vi "Dashboard Main.vi"() -> ()   [LabVIEW 2014]
uses:
  <vilib>/event_ctls.llb/eventvkey.ctl
  <vilib>/Rock Robotics/WPI/Dashboard/WPI_DashboardLogging Global.vi
  <vilib>/Rock Robotics/Network Tables/SD Read Number.vi
  <vilib>/Rock Robotics/Network Tables/SD Read Boolean.vi
  <vilib>/Rock Robotics/Network Tables/SD Write Number.vi
  <vilib>/Utility/config.llb/Write Key (String).vi
  <vilib>/Utility/config.llb/Write Key (I32).vi
  <vilib>/Utility/config.llb/NI_LVConfig.lvlib
panel:
  in  "TCP":refnum<k5>
  in  "Rec Mode":enum32{"Stop", "Record", "Playback"}(radio)
  in  "Vision":u16(ring) items=["Camera Off", "USB Camera SW", "USB Camera HW", "IP Camera"]
  out "Camera IP":string
  out "Image Message":string="Timeout in Camera Communications"
  in  "Dashboard Tab":T1(tab)
  out "Gauge":dbl(knob) scale=-0.8..0.8
  out "LatchContainerState":bool
  out "LatchLatchState":bool
  out "LatchLinkState":bool
  out "GateCylState":bool
  out "LiftCurrentHeight":dbl(slide) scale=0.0..1500.0
  out "LiftRequestedHeight":dbl(slide) scale=0.0..1500.0
  in  "ChassisSpeedDivider":dbl(slide) scale=1.25..2.0
  out "Accel":T2(graph)
  in  "Camera Settings":T3={"Frame Rate"=30, "Compression"=30, "Size"=1} {"Frame Rate" scale=1.0..30.0; "Size" items=["640x480", "320x240", "160x120"]}
  out "Mode":T4(ring)=enum."Auto Disabled"
  in  "DB Camera Config":bool
  out "fps":dbl format="%#.1g"
  out "Mbps":dbl format="%#.1g"
  out "Mbps 2":bool
  out "LiftData":T2(graph)
  in  "Test Slider":dbl(slide) scale=0.0..100.0 scale format="%#_3g"
  in  "On/Off":bool caption="Solenoid"
  in  "Test Name":u16(ring) items=["Select the test to run...", "Example Test", "-------------------------------", "List of tests is built in robot code.", "Replace with your own automated tests."]
  in  "Test Tree":string(tree)
  in  "Motor":cluster{"Value":dbl, "Enable":bool} {"Value" scale=-1.0..1.0 scale format="%#_3g"}
  out "Progress":T5 {"Test Progress" scale=0.0..100.0}
  in  "Rev/Fwd":cluster{"Forward":bool, "Reverse":bool}
  in  "Test Ring":u16(ring) items=["Monochrome", "Color"]
  in  "Listbox":i32(listbox)
  out "Tree":string(tree)
  out "Camera Image":T6(plugin-control)
  out "Boolean":bool
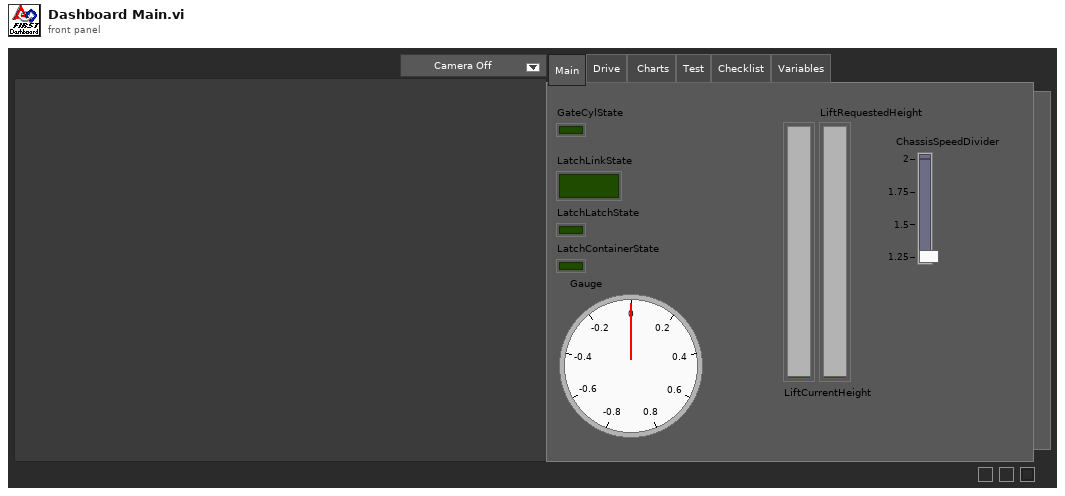
[diagram p1: front panel]
types:
  T1 = enum32{"Main", "Drive", " Charts", "Test", "Checklist", "Variables"}
  T2 = cluster{"Numeric":dbl, "Numeric":dbl, "Numeric":dbl}
  T3 = cluster{"Frame Rate":i32, "Compression":i32, "Size":u16}
  T4 = enum8{"Tele-Op Disabled", "Tele-Op Enabled", "Auto Disabled", "Auto Enabled", "Test Disabled", "Test Enabled", "Disconnected", "No Code", "E-Stop"}
  T5 = cluster{"Test Progress":u8, "Test Progress Text":string}
  T6 = typedef "IMAQ Image.ctl" = refnum<image>
  T7 = enum32{"Drive", "Basic", "Custom", "Test", "Checklist", "Variables"}
  T8 = typedef "Image Type" = u32
  T9 = cluster{"Camera Image":refnum<vi>, "Dashboard Tab":refnum<vi>, "Boolean":refnum<vi>, "Vision":refnum<vi>, "Rec Mode":refnum<vi>, "Test Slider":refnum<vi>, "On/Off ":refnum<vi>, "Test Ring":refnum<vi>, "Rev/Fwd":refnum<vi>, "Test Name":refnum<vi>, "Motor":refnum<vi>, "Progress":refnum<vi>, "CheckList":refnum<vi>, "Tree":refnum<vi>, "Test Tree":refnum<vi>}
  T10 = cluster{"Error Strings":string, "Disable Counts":cluster{u16, u16}, "Rail Faults":cluster{u16, u16, u16}, "Robot IP":string, "DB Mode":u8, "Event Info":cluster{"Name":string, "Type":u8, "Number":u16, "Replay":u8}, "Camera Addr":string}
  T11 = cluster{"Storage":cluster{"Disk Free":u64, "RAM Block":u32, "RAM free":u32}, "CPU Utilization":cluster{"CPU % ISR":sgl, "CPU % Time Crit":sgl, "CPU % Timed Str":sgl, "CPU % High":sgl, "CPU % Above":sgl, "CPU % Normal":sgl, "CPU % Low":sgl}, "CAN":cluster{"% Bus Utilization":sgl, "Bus Off Cnt":u32, "TX_FIFO Full Cnt":u32, "Receive Error Cnt":u8, "Transmit Error Cnt":u8}, "HID":cluster{"HID Outputs":u32, "Rumble Low":u16, "Rumble High":u16}[]}
  T12 = cluster{"Status bits":cluster{"Test Mode":bool, "Autonomous":bool, "Enabled":bool, "Code Start":bool, "Brownout":bool, "Reserved 2":bool, "Reserved 3":bool, "E-Stop":bool}, "Code Trace":cluster{"Disabled":bool, "TeleOp":bool, "Auto":bool, "Test":bool}, "Controller Type":enum16{"unknown", "cRIO", "roboRio"}, "Code?":enum16{"unknown", "noCode", "code"}, "Battery V":dbl}
  T13 = cluster{"Control Bits":cluster{"TestMode":bool, "Autonomous":bool, "Enabled":bool, "FMS Present":bool, bool, bool, bool, "E-Stop":bool}, "Team Station ":u8, "Countdown":sgl, "Joystick Values":cluster{"Axes":dbl[], "Buttons":bool[], "POVs":i16[]}[]}
  T14 = typedef "NI_LVConfig.lvlib/Config Data RefNum.ctl" = refnum<k1>
  T15 = cluster{"Operation":enum16{"Update", "Clear"}, "Color Box":u32}[]
  T16 = typedef "eventvkey.ctl" = enum16{"ASCII", "Enter", "Return", "Shift", "Ctrl", "Alt", "Cmd", "Opt", "Caps", "NumLock", "Clear", "Break", "Up", "Down", "Left", "Right", "Insert", "Delete", "Home", "End", "PageUp", "PageDown", "Escape", "Help", "Pause", "ScrollLock", "F1", "F2", "F3", "F4", "F5", "F6", "F7", "F8", "F9", "F10", "F11", "F12", "F13", "F14", "F15", "F16", "F17", "F18", "F19", "F20", "F21", "F22", "F23", "F24", "Play", "VolumeUp", "VolumeDown", "Mute", "Two Byte Char"}
  T17 = cluster{"Image Size":bool, "Image Type":bool, "Pixel Value":bool, "ROI Information":bool, "Zoom Factor":bool}
  T18 = enum8{"Enabled", "Disabled", "Disabled and Grayed Out"}
  T19 = cluster{"Operation":enum16{"Update", "Clear"}, "Color Box":u32}
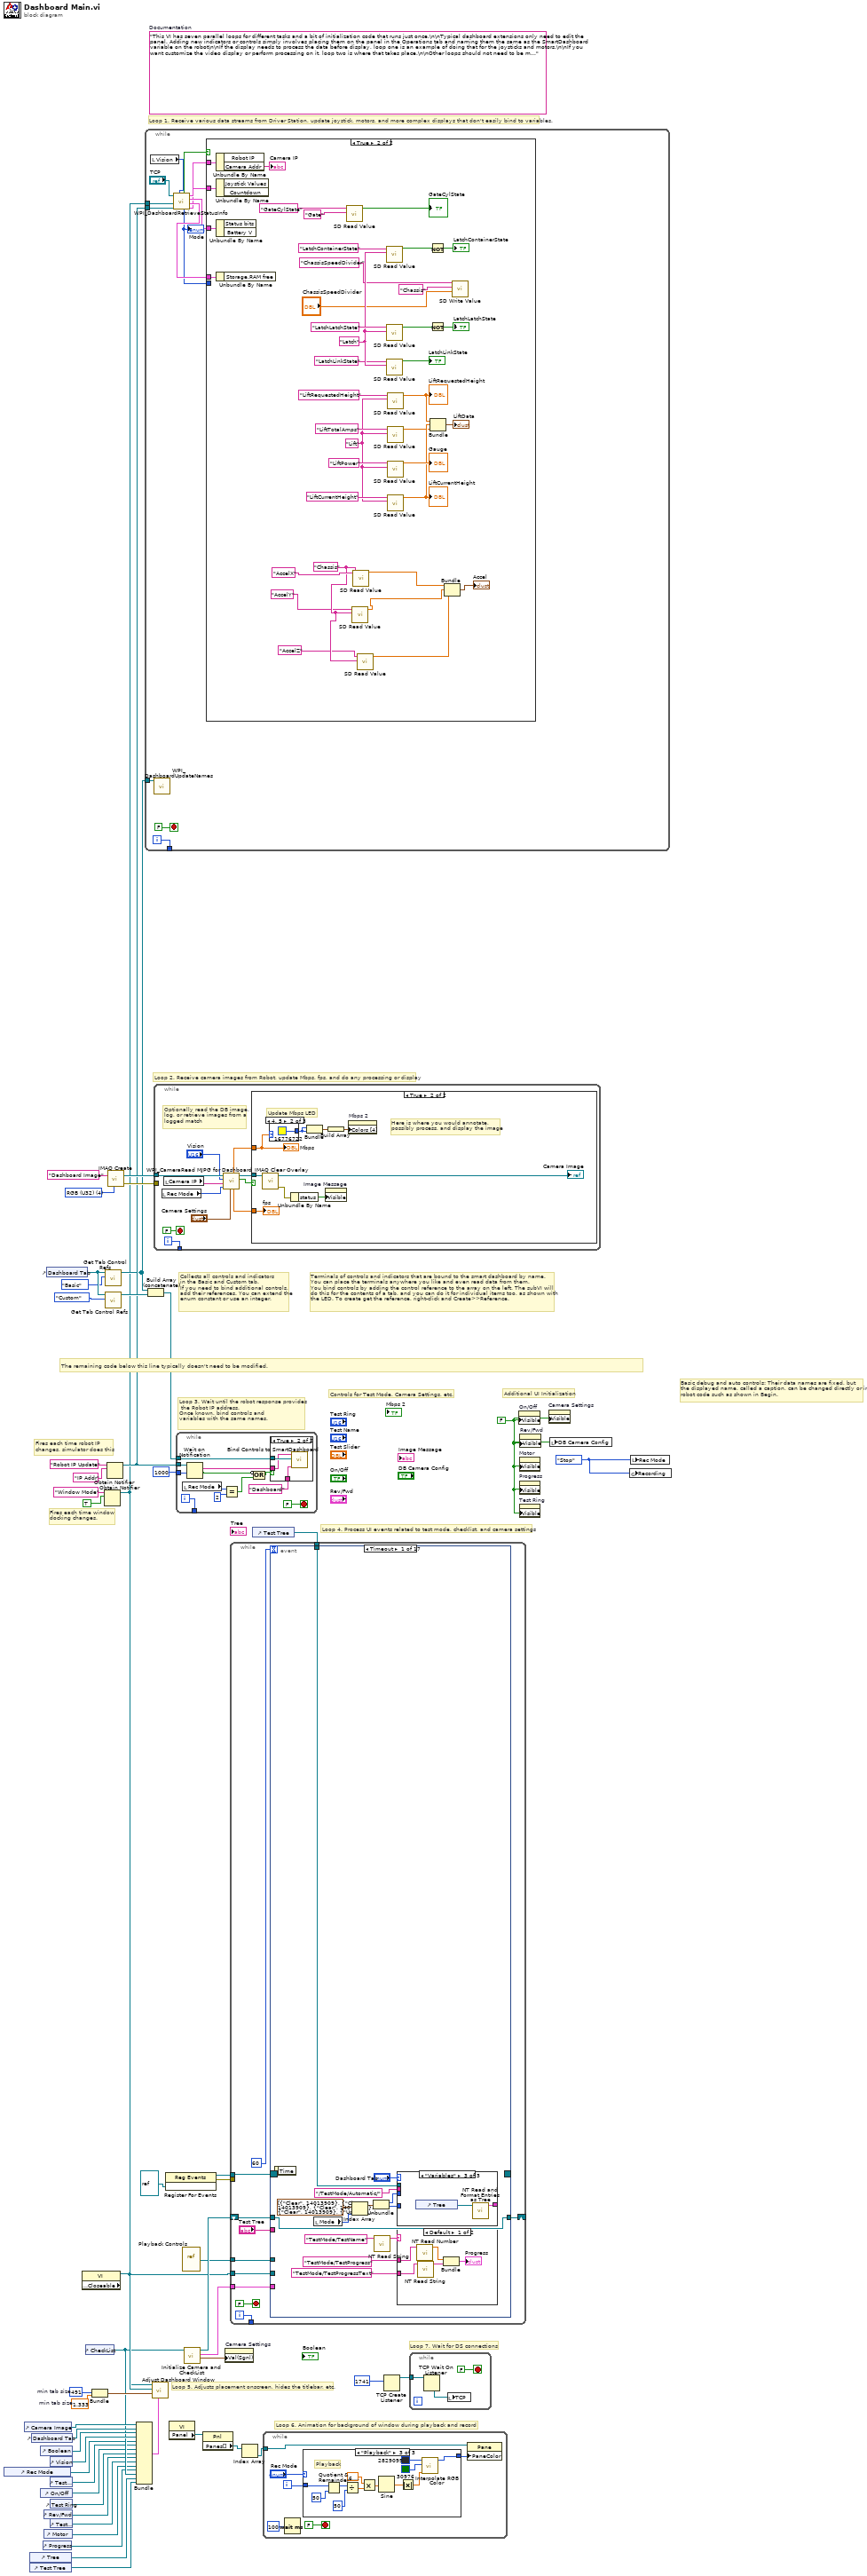
[diagram p0: block diagram]
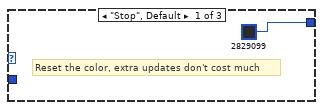
[diagram p3: hidden frame]
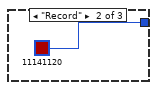
[diagram p4: hidden frame]
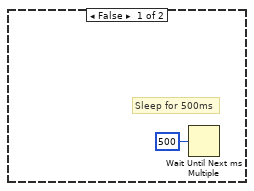
[diagram p6: hidden frame]
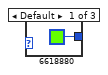
[diagram p7: hidden frame]
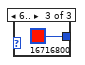
[diagram p8: hidden frame]
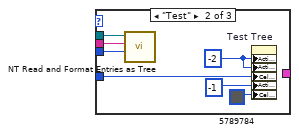
[diagram p10: hidden frame]
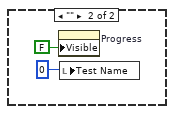
[diagram p11: hidden frame]
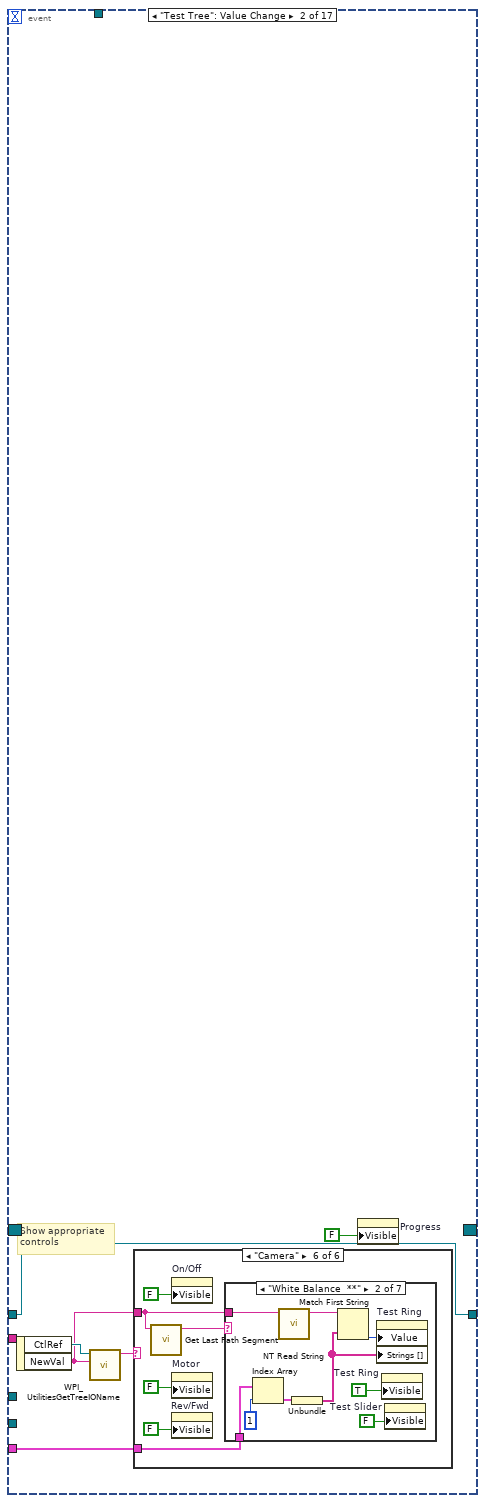
[diagram p12: hidden frame]
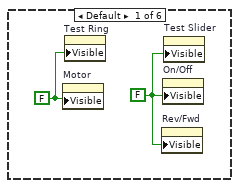
[diagram p13: hidden frame]
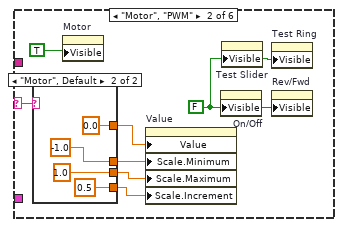
[diagram p14: hidden frame]
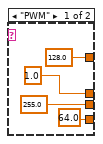
[diagram p15: hidden frame]
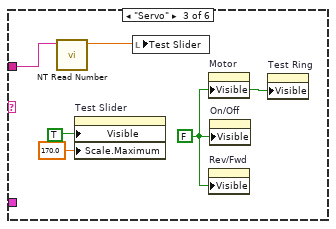
[diagram p16: hidden frame]
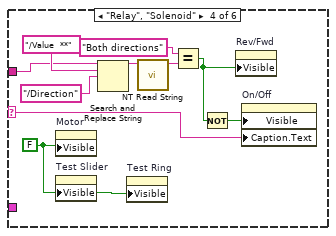
[diagram p17: hidden frame]
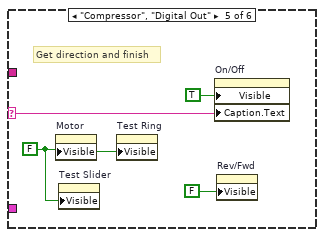
[diagram p18: hidden frame]
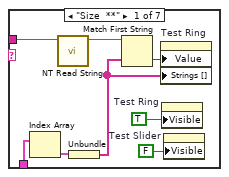
[diagram p19: hidden frame]
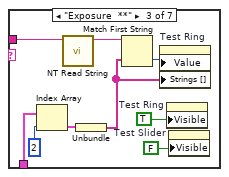
[diagram p20: hidden frame]
diagram:
  w24 = 491  # min tab size
  w23 = 1.333  # min tab size
  w32 = enum32{"Stop", "Record", "Playback"}."Stop" ("Rec Mode")
  w6 = FALSE ("Visible")
  (unwired) "This VI has seven parallel loops for different tasks and a bit of initialization code that runs just once.\n\nTypical dashboard extensions only need to edit the panel. Adding new indicators or controls simply involves placing them on the panel in the Operations tab and naming them the same as the SmartDashboard variable on the robot\n\nIf the display needs to process the data before display, loop one is an example of doing that for the joysticks and motors.\n\nIf you want customize the video display or perform processing on it, loop two is where that takes place.\n\nOther loops should not need to be modified. They are pretty standard, and document the task they perform."  # Documentation
  w52 = T8 4 items=["Grayscale (U8)", "Grayscale (I16)", "Grayscale (SGL)", "Complex (CSG)", "RGB (U32)", "HSL (U32)", "RGB (U64)"] ("Image Type")
  # "Loop 7. Wait for DS connections"
  # "Basic debug and auto controls: Their data names are fixed, but\nthe displayed name, called a caption, can be changed directly or in\nrobot code such as shown in Begin."
  # "Controls for Test Mode, Camera Settings, etc."
  # "Additional UI Initialization"
  # "Loop 6. Animation for background of window during playback and record"
  # "Fires each time robot IP\nchanges, simulator does this"
  # "Fires each time window\ndocking changes."
  # "Collects all controls and indicators\nin the Basic and Custom tab.\nIf you need to bind additional controls,\nadd their references. You can extend the\nenum constant or use an integer."
  # "The remaining code below this line typically doesn't need to be modified."
  # "Loop 4. Process UI events related to test mode, checklist, and camera settings"
  # "Terminals of controls and indicators that are bound to the smart dashboard by name.\nYou can place the terminals anywhere you like and even read data from them.\nYou bind controls by adding the control reference to the array on the left. The subVI will\ndo this for the contents of a tab, and you can do it for individual items too, as shown with\nthe LED. To create get the reference, right-click and Create>>Reference."
  # "Loop 3. Wait until the robot response provides\n the Robot IP address.\nOnce known, bind controls and\nvariables with the same names."
  # "Loop 5. Adjusts placement onscreen, hides the titlebar, etc."
  # "Loop 1. Receive various data streams from Driver Station, update joystick, motors, and more complex displays that don't easily bind to variables."
  # "Loop 2. Receive camera images from Robot, update Mbps, fps, and do any processing or display"
  n1 = control-ref of="Rec Mode"() -> (w12:refnum<vi>)
  n2 = control-ref of="Camera Image"() -> (w27:refnum<vi>)
  n3 = control-ref of="Tree"() -> (w16:refnum<vi>)
  n4 = control-ref of="Test Tree"() -> (w15:refnum<vi>)
  n5 = control-ref of="Dashboard Tab"() -> (w26:refnum<vi>)
  n6 = control-ref of="Boolean"() -> (w21:refnum<vi>)
  n7 = control-ref of="On/Off"() -> (w10:refnum<vi>)
  n8 = control-ref of="Progress"() -> (w7:refnum<vi>)
  n9 = control-ref of="Rev/Fwd"() -> (w8:refnum<vi>)
  n10 = control-ref of="Motor"() -> (w13:refnum<vi>)
  n11 = control-ref of="Dashboard Tab"() -> (w30:refnum<vi>)
  n12 = control-ref of="Test Slider"() -> (w11:refnum<vi>)
  n13 = control-ref of="Vision"() -> (w25:refnum<vi>)
  n14 = control-ref of="Test Ring"() -> (w9:refnum<vi>)
  n15 = control-ref of="Test Name"() -> (w14:refnum<vi>)
  n16 = property class="VI" props=["Front Panel.Closeable"]() -> (reference out=w31:refnum<vi>)  [unwired: 2 in, 2 out]
  n17 = control-ref of="CheckList"() -> (w17:refnum<vi>)
  n18 = Bundle("min tab size"=w24, "min tab size"=w23) -> (w22:cluster{"min tab size":i32, "min tab size":dbl})  [unwired: 1 in]
  n19 = Obtain Notifier(name (unnamed)="Window Mode", notification data type=TRUE) -> (notifier out=w3:refnum<notifier>)  [unwired: 2 in, 2 out]
  n20 = call <vilib>:"Get Tab Control Refs.vi"("Page Index"=T7."Basic" ("Dashboard Tab"), "TabControl in"=w30) -> ("ControlsOnPage"=w4:refnum<vi>[])  [unwired: 9 in]
  n21 = call <vilib>:"Get Tab Control Refs.vi"("Page Index"=T7."Custom" ("Dashboard Tab"), "TabControl in"=w30) -> ("ControlsOnPage"=w29:refnum<vi>[])  [unwired: 9 in]
  n22 = Obtain Notifier(name (unnamed)="Robot IP Update", notification data type="IP Addr" ("name (unnamed)")) -> (notifier out=w5:refnum<notifier>)  [unwired: 2 in, 2 out]
  n23 = call "IMAQ Create"("Image Name"="Dashboard Image", "Image Type"=w52) -> ("New Image"=w50:T6, "error out"=w49:errorcluster)  [unwired: 2 in, 1 out]
  n24 = Bundle("Camera Image"=w27, "Dashboard Tab"=w26, "Boolean"=w21, "Vision"=w25, "Rec Mode"=w12, "Test Slider"=w11, "On/Off"=w10, "Test Ring"=w9, "Rev/Fwd"=w8, "Test Name"=w14, "Motor"=w13, "Progress"=w7, "CheckList"=w17, "Tree"=w16, "Test Tree"=w15) -> (w18:T9)  [unwired: 1 in]
  n25 = while {
    tunnel: [w64] -> _
    tunnel: w5 -> [w58]
    tunnel: w4 -> [w57]
    tunnel: w3 -> [w53]
    i -> [w64]
    stop <- FALSE stop-if-true
    n26 = local read "Vision"() -> (w55:u16)
    n27 = call <vilib>:"WPI_DashboardUpdateNames.vi"("Controls on Tab"=w57) -> ()  [unwired: 11 in]
    n28 = call <vilib>:"WPI_DashboardRetrieveStatusInfo.vi"("Vision"=w55, "Binding Refnum"=w58, "Window Mode Notifier"=w53, "TCP Cnx"="TCP") -> ("Power and Errors"=w59:T10, "Robot Metrics"=w62:T11, "Status Info"=w63:T12, "Control Info"=w60:T13, "Robot Mode"=w56:T4, "Process?"=w61:bool)  [unwired: 2 in]
    "Mode" <- w56
    n29 = case shown="True" w61 {
      tunnel: w63 -> [_ w103]
      tunnel: w62 -> [_ w102]
      tunnel: w60 -> [_ w101]
      tunnel: w59 -> [_ w100]
      tunnel: w56 -> [_ _]
      frame False {
      }
      frame True {
        w72 = "Chassis" ("Table Prefix")
        w90 = "Latch"
        w75 = "Lift" ("Table Prefix")
        n30 = Unbundle By Name(w100) -> ("Camera Addr"=→"Camera IP":string)  [unwired: 1 out]
        n31 = Unbundle By Name(w101) -> ()  [unwired: 2 out]
        n32 = Unbundle By Name(w103) -> ()  [unwired: 2 out]
        n33 = Unbundle By Name(w102) -> ()  [unwired: 1 out]
        n34 = call-poly <vilib>:"SD Read Value.vi"("Table Prefix"="Gate", "Name"="GateCylState") -> ("Boolean"=→"GateCylState":bool)  [unwired: 7 in, 2 out]
        n35 = call-poly <vilib>:"SD Read Value.vi"("Table Prefix"=w72, "Name"="AccelY") -> ("Numeric"=w67:dbl)  [unwired: 7 in, 2 out]
        n36 = call-poly <vilib>:"SD Read Value.vi"("Table Prefix"=w72, "Name"="AccelX") -> ("Numeric"=w68:dbl)  [unwired: 7 in, 2 out]
        n37 = call-poly <vilib>:"SD Read Value.vi"("Table Prefix"=w72, "Name"="AccelZ") -> ("Numeric"=w66:dbl)  [unwired: 7 in, 2 out]
        n38 = call-poly <vilib>:"SD Read Value.vi"("Table Prefix"=w90, "Name"="LatchContainerState") -> ("Boolean"=w87:bool)  [unwired: 7 in, 2 out]
        n39 = call-poly <vilib>:"SD Read Value.vi"("Table Prefix"=w90, "Name"="LatchLatchState") -> ("Boolean"=w85:bool)  [unwired: 7 in, 2 out]
        n40 = call-poly <vilib>:"SD Read Value.vi"("Table Prefix"=w90, "Name"="LatchLinkState") -> ("Boolean"=→"LatchLinkState":bool)  [unwired: 7 in, 2 out]
        n41 = call-poly <vilib>:"SD Read Value.vi"("Table Prefix"=w75, "Name"="LiftRequestedHeight") -> ("Numeric"=w79:dbl)  [unwired: 7 in, 2 out]
        "LiftRequestedHeight" <- w79
        n42 = call-poly <vilib>:"SD Read Value.vi"("Table Prefix"=w75, "Name"="LiftTotalAmps") -> ("Numeric"=w74:dbl)  [unwired: 7 in, 2 out]
        n43 = call-poly <vilib>:"SD Read Value.vi"("Table Prefix"=w75, "Name"="LiftPower") -> ("Numeric"=→"Gauge":dbl)  [unwired: 7 in, 2 out]
        n44 = call-poly <vilib>:"SD Read Value.vi"("Table Prefix"=w75, "Name"="LiftCurrentHeight") -> ("Numeric"=w78:dbl)  [unwired: 7 in, 2 out]
        "LiftCurrentHeight" <- w78
        n45 = Not(x=w87) -> (.not. x?=→"LatchContainerState":bool)
        n46 = Not(x=w85) -> (.not. x?=→"LatchLatchState":bool)
        n47 = Bundle("Numeric"=w79, "Numeric"=w78, "Numeric"=w74) -> (→"LiftData":T2)  [unwired: 1 in]
        n48 = Bundle("Numeric"=w68, "Numeric"=w67, "Numeric"=w66) -> (→"Accel":T2)  [unwired: 1 in]
        n49 = call-poly <vilib>:"SD Write Value.vi"("Numeric"="ChassisSpeedDivider", "Table Prefix"="Chassis", "Name"="ChassisSpeedDivider") -> ()  [unwired: 7 in, 2 out]
      }
    }
  }
  n50 = Build Array (concatenate)(w4, w29) -> (w28:refnum<vi>[])
  n51 = call "Adjust Dashboard Window.vi"("Sizing Refnums"=w18, "Size Constraints"=w22, "VI"=w31, "Notifier in"=w3) -> ()  [unwired: 8 in]
  n52 = while {
    tunnel: w50 -> [w112]
    tunnel: w49 -> [_]
    tunnel: [w113] -> _
    i -> [w113]
    stop <- FALSE stop-if-true
    # "Optionally read the DB image,\nlog, or retrieve images from a\nlogged match"
    n53 = local read "Rec Mode"() -> (w106:enum32{"Stop", "Record", "Playback"})
    n54 = local read "Camera IP"() -> (w104:string)
    n55 = call <vilib>:"WPI_CameraRead MJPG for Dashboard.vi"("Camera Settings"="Camera Settings", "Rec Mode"=w106, "Camera IP"=w104, "Camera Mode"="Vision", "Refnum in"=w112) -> ("Active"=w110:bool, "Refnum out"=w111:T6, "FPS"=w109:dbl, "Bandwidth (Mbps)"=w108:dbl)  [unwired: 3 in]
    n56 = case shown="True" w110 {
      tunnel: w111 -> [_ w119]
      tunnel: w108 -> [_ w118]
      tunnel: w109 -> [_ w116]
      frame False {
        # "Sleep for 500ms"
        n57 = Wait Until Next ms Multiple(millisecond multiple=u32 500) -> ()  [unwired: 1 out]
      }
      frame True {
        # "Here is where you would annotate,\npossibly process, and display the image"
        # "Update Mbps LED"
        n58 = call "IMAQ Clear Overlay"("Image"=w119) -> ("error out"=w123:errorcluster, "Image Out"=→"Camera Image":T6)  [unwired: 2 in, 7 out]
        n59 = case shown="4, 5" w118 {
          tunnel: [u32 6618880 ("Color Box") u32 16776722 ("Color Box") u32 16716800 ("Color Box")] -> w120
          frame Default {
          }
          frame 4, 5 {
          }
          frame 6.. {
          }
        }
        n60 = Unbundle By Name(w123) -> ("status"=w124:bool)
        n61 = Bundle("Color Box"=w120, "Color Box"=w120) -> (w122:cluster{"Color Box":u32, "Color Box":u32})  [unwired: 1 out]
        n62 = property on="Image Message" class="Str"("Visible"=w124) -> ()  [unwired: 2 in, 2 out]
        n63 = Build Array(w122) -> (w121:cluster{"Color Box":u32, "Color Box":u32}[])
        n64 = property on="Mbps 2" class="Bool (strict)"("Colors [4]"=w121) -> ()  [unwired: 2 in, 2 out]
        "Mbps" <- w118
        "fps" <- w116
      }
    }
  }
  n65 = register-events(refnum<vi> refnum) -> (reference out=w36:refnum<event-registration>, error out=w35:errorcluster)  [unwired: 2 in]
  n66 = property class="VI"() -> ("Panel"=w39:refnum<vi>)  [unwired: 2 in, 2 out]
  n67 = while {
    tunnel: w28 -> [w139]
    tunnel: w5 -> [w137]
    tunnel: [w135] -> _
    tunnel: u32 1000 ("milliseconds to wait") -> [w134]
    i -> [w135]
    stop <- FALSE stop-if-true
    n68 = local read "Rec Mode"() -> (w130:enum32{"Stop", "Record", "Playback"})
    n69 = Wait on Notification(notifier=w137, timeout in ms (-1)=w134) -> (notification=w136:string, timed out?=w132:bool)  [unwired: 2 in, 2 out]
    n70 = Equal?(x=w130, y=u16 2 ("Rec Mode")) -> (x = y?=w131:bool)
    n71 = Compound Arithmetic op=OR(invert w132, w131) -> (w133:bool)
    n72 = case shown="True" w133 {
      tunnel: w139 -> [_ w142]
      tunnel: w136 -> [_ w141]
      tunnel: "Dashboard" -> [_ w140]
      frame False {
      }
      frame True {
        n73 = call <vilib>:"Bind Controls to SmartDashboard.vi"("Client Name"=w140, "Bound Control Refs"=w142, "Server IP Address"=w141) -> ()  [unwired: 9 in]
      }
    }
  }
  n74 = vi-ref "Playback Controls.vi"() -> (w37:refnum<vi>)
  n75 = call "Initialize Camera and CheckList.vi"("ListBox in"=w17) -> ("Cluster"=w43:cluster{"value":i32, "value":i32, "index":i32}, "Array"=w44:cluster{string[]}[], "File Refnum"=w42:T14)  [unwired: 8 in]
  n76 = property class="Pnl"(reference=w39) -> ("Panes[]"=w40:refnum<vi>[])  [unwired: 1 in, 2 out]
  n77 = property on="Camera Settings" class="Clust (strict)"("Val(Sgnl)"=w43) -> ()  [unwired: 2 in, 2 out]
  n78 = Index Array(array=w40) -> (element=w38:refnum<vi>)  [unwired: 1 in]
  n79 = control-ref of="Test Tree"() -> (w41:refnum<vi>)
  n80 = while {
    tunnel: w44 -> [w150]
    shift-right: [w149] -> _
    shift-left: w42 -> [w148]
    tunnel: [w147] -> _
    tunnel: w41 -> [w146]
    tunnel: w37 -> [w145]
    tunnel: w36 -> [w144]
    tunnel: w35 -> [_]
    tunnel: w31 -> [w143]
    i -> [w147]
    stop <- FALSE stop-if-true
    n81 = event shown="[0] Timeout" {
      selector: w144 -> [_ _ _ _ _ _ _ _ _ _ _ _ _ _ _ _ _]
      dyn-events: [_ _ _ _ _ _ _ _ _ _ _ _ _ w388 _ _ _] -> _
      timeout: u32 60 ("milliseconds to wait") -> [_ _ _ _ _ _ _ _ _ _ _ _ _ _ _ _ _]
      tunnel: w146 -> [w162 _ _ _ _ _ _ _ _ _ _ _ _ _ _ _ _]
      tunnel: "Test Tree" -> [_ _ _ _ _ _ _ _ w357 w365 w367 w371 w379 _ _ _ _]
      tunnel: w150 -> [_ w184 _ _ _ _ w321 w351 _ _ _ _ _ _ _ _ _]
      tunnel: [w158 w183 w282 w287 w295 w307 w320 w344 w356 w363 w366 w370 w378 w390 w404 w405 w415] -> w149
      tunnel: w148 -> [w158 w183 w282 w287 w295 w307 w319 w344 w356 w363 w366 w370 w378 w390 w404 w405 w415]
      tunnel: w145 -> [_ _ _ _ _ _ _ _ _ _ _ _ _ w391 _ w408 _]
      tunnel: w143 -> [_ _ _ _ _ _ _ _ _ _ _ _ _ w386 _ _ _]
      event Timeout {
        n82 = event-data() -> ()  [unwired: 1 in, 1 out]
        n83 = local read "Mode"() -> (w161:T4)
        n84 = Index Array(array=T15 [{"Operation"=enum."Clear", "Color Box"=14013909}, {"Operation"=enum."Clear", "Color Box"=14013909}, {"Operation"=enum."Clear", "Color Box"=14013909}, {"Operation"=enum."Clear", "Color Box"=14013909}, {"Operation"=enum."Update", "Color Box"=14013909}, {"Operation"=enum."Update", "Color Box"=16777215}, {"Operation"=enum."Clear", "Color Box"=14013909}, {"Operation"=enum."Clear", "Color Box"=14013909}, {"Operation"=enum."Clear", "Color Box"=14013909}], index=w161) -> (element=w156:T19)
        n85 = Unbundle(w156) -> ("Operation"=w155:enum16{"Update", "Clear"}, "Color Box"=w154:u32)
        n86 = call <vilib>:"NT Read String.vi"("Name"="TestMode/TestName") -> ("String"=w165:string)  [unwired: 9 in, 1 out]
        n87 = case shown="\"Variables\"" "Dashboard Tab" {
          tunnel: w162 -> [_ w173 _]
          tunnel: "/TestMode/Automatic/" ("Name Pattern") -> [_ w172 _]
          tunnel: w155 -> [_ w171 _]
          tunnel: [_ _ w175] -> _
          tunnel: w154 -> [_ w167 _]
          frame "Main", Default {
          }
          frame "Test" {
            w170 = -2 ("Active Item:Row Number")
            n88 = call <vilib>:"NT Read and Format Entries as Tree.vi"("Operation"=w171, "Name Pattern"=w172, "Tree Refnum"=w173) -> ()  [unwired: 7 in, 2 out]
            n89 = property on="Test Tree" class="Tree (strict)"("Active Item Row Number"=w170, "ActiveColNum"=w170, "CellBG"=w167, "Active Item Row Number"=-1 ("Active Item:Row Number"), "CellBG"=u32 5789784 ("Color Box")) -> ()  [unwired: 2 in, 2 out]
          }
          frame "Variables" {
            n90 = control-ref of="Tree"() -> (w174:refnum<vi>)
            n91 = call <vilib>:"NT Read and Format Entries as Tree.vi"("Tree Refnum"=w174) -> ("Formatted Strings"=w175:cluster{"Name":string, "Value":string}[])  [unwired: 9 in, 1 out]
          }
        }
        n92 = case shown="Default" w165 {
          tunnel: "TestMode/TestProgress" ("Name") -> [w177 _]
          tunnel: "TestMode/TestProgressText" ("Name") -> [w176 _]
          frame Default {
            n93 = call <vilib>:"NT Read Number.vi"("Name"=w177) -> ("Numeric"=w178:dbl)  [unwired: 9 in, 1 out]
            n94 = call <vilib>:"NT Read String.vi"("Name"=w176) -> ("String"=w179:string)  [unwired: 9 in, 1 out]
            n95 = Bundle("Numeric"=w178, "String"=w179) -> (→"Progress":cluster{"Numeric":dbl, "String":string})  [unwired: 1 in]
          }
          frame "" {
            n96 = property on="Progress" class="Clust (strict)"("Visible"=FALSE) -> ()  [unwired: 2 in, 2 out]
            n97 = local write "Test Name"(u16 0) -> ()
          }
        }
      }
      event "Test Tree": Value Change {
        # "Show appropriate\ncontrols"
        n98 = event-data() -> ("CtlRef"=w187:refnum<vi>, "NewVal"=w185:string)  [unwired: 1 in]
        n99 = call <vilib>:"WPI_UtilitiesGetTreeIOName.vi"("NewVal"=w185, "TreeControl in"=w187) -> ("I/O Name"=w188:string)  [unwired: 9 in]
        n100 = case shown="\"Camera\"" w188 {
          selector: w188 -> [_ w195 _ w213 w222 _]
          tunnel: w185 -> [_ _ w210 w212 _ w229]
          tunnel: w184 -> [_ _ _ _ _ w228]
          frame Default {
            w190 = FALSE ("Visible")
            w189 = FALSE ("Visible")
            n101 = property on="Motor" class="Clust (strict)"("Visible"=w189) -> ()  [unwired: 2 in, 2 out]
            n102 = property on="Test Ring" class="Ring (strict)"("Visible"=w189) -> ()  [unwired: 2 in, 2 out]
            n103 = property on="Rev/Fwd" class="Clust (strict)"("Visible"=w190) -> ()  [unwired: 2 in, 2 out]
            n104 = property on="On/Off" class="Bool (strict)"("Visible"=w190) -> ()  [unwired: 2 in, 2 out]
            n105 = property on="Test Slider" class="Slide (strict)"("Visible"=w190) -> ()  [unwired: 2 in, 2 out]
          }
          frame "Motor", "PWM" {
            w196 = FALSE ("Visible")
            n106 = case shown="\"Motor\", Default" w195 {
              tunnel: [1.0 ("Value") -1.0 ("Value")] -> w194
              tunnel: [255.0 ("Value") 1.0 ("Value")] -> w193
              tunnel: [128.0 ("Value") 0.0 ("Value")] -> w192
              tunnel: [64.0 ("Value") 0.5 ("Value")] -> w191
              frame "PWM" {
              }
              frame "Motor", Default {
              }
            }
            n107 = property on="Motor" class="Clust (strict)"("Visible"=TRUE) -> ()  [unwired: 2 in, 2 out]
            n108 = property on="Value" class="Slide (strict)"("Value"=w192, "Scale.Minimum"=w194, "Scale.Maximum"=w193, "Scale.Increment"=w191) -> ()  [unwired: 2 in, 2 out]
            n109 = property on="On/Off" class="Bool (strict)"("Visible"=w196) -> ()  [unwired: 2 in, 2 out]
            n110 = property on="Test Slider" class="Slide (strict)"("Visible"=w196) -> ()  [unwired: 2 in, 2 out]
            n111 = property on="Test Ring" class="Ring (strict)"("Visible"=w196) -> ()  [unwired: 2 in, 2 out]
            n112 = property on="Rev/Fwd" class="Clust (strict)"("Visible"=w196) -> ()  [unwired: 2 in, 2 out]
          }
          frame "Servo" {
            w208 = FALSE ("Visible")
            n113 = call <vilib>:"NT Read Number.vi"("Name"=w210) -> ("Numeric"=w209:dbl)  [unwired: 9 in, 1 out]
            n114 = property on="Test Slider" class="Slide (strict)"("Visible"=TRUE, "Scale.Maximum"=170.0 ("Scale.Range:Maximum")) -> ()  [unwired: 2 in, 2 out]
            n115 = local write "Test Slider"(w209) -> ()
            n116 = property on="Motor" class="Clust (strict)"("Visible"=w208) -> ()  [unwired: 2 in, 2 out]
            n117 = property on="Rev/Fwd" class="Clust (strict)"("Visible"=w208) -> ()  [unwired: 2 in, 2 out]
            n118 = property on="On/Off" class="Bool (strict)"("Visible"=w208) -> ()  [unwired: 2 in, 2 out]
            n119 = property on="Test Ring" class="Ring (strict)"("Visible"=w208) -> ()  [unwired: 2 in, 2 out]
          }
          frame "Relay", "Solenoid" {
            w211 = FALSE ("Visible")
            n120 = property on="Motor" class="Clust (strict)"("Visible"=w211) -> ()  [unwired: 2 in, 2 out]
            n121 = property on="Test Slider" class="Slide (strict)"("Visible"=w211) -> ()  [unwired: 2 in, 2 out]
            n122 = Search and Replace String(input string=w212, search string="/Value  **", replace string="/Direction") -> (result string=w218:string)  [unwired: 5 in, 3 out]
            n123 = property on="Test Ring" class="Ring (strict)"("Visible"=w211) -> ()  [unwired: 2 in, 2 out]
            n124 = call <vilib>:"NT Read String.vi"("Name"=w218) -> ("String"=w216:string)  [unwired: 9 in, 1 out]
            n125 = Equal?(x="Both directions", y=w216) -> (x = y?=w214:bool)
            n126 = Not(x=w214) -> (.not. x?=w215:bool)
            n127 = property on="Rev/Fwd" class="Clust (strict)"("Visible"=w214) -> ()  [unwired: 2 in, 2 out]
            n128 = property on="On/Off" class="Bool (strict)"("Visible"=w215, "Caption.Text"=w213) -> ()  [unwired: 2 in, 2 out]
          }
          frame "Compressor", "Digital Out" {
            w221 = FALSE ("Visible")
            # "Get direction and finish"
            n129 = property on="Motor" class="Clust (strict)"("Visible"=w221) -> ()  [unwired: 2 in, 2 out]
            n130 = property on="Test Slider" class="Slide (strict)"("Visible"=w221) -> ()  [unwired: 2 in, 2 out]
            n131 = property on="Test Ring" class="Ring (strict)"("Visible"=w221) -> ()  [unwired: 2 in, 2 out]
            n132 = property on="On/Off" class="Bool (strict)"("Visible"=TRUE, "Caption.Text"=w222) -> ()  [unwired: 2 in, 2 out]
            n133 = property on="Rev/Fwd" class="Clust (strict)"("Visible"=FALSE) -> ()  [unwired: 2 in, 2 out]
          }
          frame "Camera" {
            n134 = call <vilib>:"Get Last Path Segment.vi"("String in"=w229) -> ("String out"=w230:string)  [unwired: 10 in]
            n135 = property on="On/Off" class="Bool (strict)"("Visible"=FALSE) -> ()  [unwired: 2 in, 2 out]
            n136 = property on="Motor" class="Clust (strict)"("Visible"=FALSE) -> ()  [unwired: 2 in, 2 out]
            n137 = property on="Rev/Fwd" class="Clust (strict)"("Visible"=FALSE) -> ()  [unwired: 2 in, 2 out]
            n138 = case shown="\"White Balance  **\"" w230 {
              tunnel: w229 -> [w236 w245 w254 w263 w272 _ w278]
              tunnel: w228 -> [w234 w242 w251 w260 w269 _ _]
              frame "Size  **" {
                n139 = Index Array(array=w234) -> (element=w233:cluster{string[]})  [unwired: 1 in]
                n140 = call <vilib>:"NT Read String.vi"("Name"=w236) -> ("String"=w235:string)  [unwired: 9 in, 1 out]
                n141 = Unbundle(w233) -> (w231:string[])
                n142 = Match First String(2:w231, 3:w235) -> (0:w232:i32)  [unwired: 1 out]
                n143 = property on="Test Ring" class="Ring (strict)"("Value"=w232, "Strings []"=w231) -> ()  [unwired: 2 in, 2 out]
                n144 = property on="Test Ring" class="Ring (strict)"("Visible"=TRUE) -> ()  [unwired: 2 in, 2 out]
                n145 = property on="Test Slider" class="Slide (strict)"("Visible"=FALSE) -> ()  [unwired: 2 in, 2 out]
              }
              frame "White Balance  **" {
                n146 = Index Array(array=w242, index=1) -> (element=w243:cluster{string[]})
                n147 = call <vilib>:"NT Read String.vi"("Name"=w245) -> ("String"=w244:string)  [unwired: 9 in, 1 out]
                n148 = Unbundle(w243) -> (w240:string[])
                n149 = Match First String(2:w240, 3:w244) -> (0:w239:i32)  [unwired: 1 out]
                n150 = property on="Test Ring" class="Ring (strict)"("Value"=w239, "Strings []"=w240) -> ()  [unwired: 2 in, 2 out]
                n151 = property on="Test Ring" class="Ring (strict)"("Visible"=TRUE) -> ()  [unwired: 2 in, 2 out]
                n152 = property on="Test Slider" class="Slide (strict)"("Visible"=FALSE) -> ()  [unwired: 2 in, 2 out]
              }
              frame "Exposure  **" {
                n153 = Index Array(array=w251, index=2) -> (element=w252:cluster{string[]})
                n154 = call <vilib>:"NT Read String.vi"("Name"=w254) -> ("String"=w253:string)  [unwired: 9 in, 1 out]
                n155 = Unbundle(w252) -> (w248:string[])
                n156 = Match First String(2:w248, 3:w253) -> (0:w249:i32)  [unwired: 1 out]
                n157 = property on="Test Ring" class="Ring (strict)"("Value"=w249, "Strings []"=w248) -> ()  [unwired: 2 in, 2 out]
                n158 = property on="Test Ring" class="Ring (strict)"("Visible"=TRUE) -> ()  [unwired: 2 in, 2 out]
                n159 = property on="Test Slider" class="Slide (strict)"("Visible"=FALSE) -> ()  [unwired: 2 in, 2 out]
              }
              frame "Exposure Priority  **" {
                n160 = Index Array(array=w260, index=3) -> (element=w261:cluster{string[]})
                n161 = call <vilib>:"NT Read String.vi"("Name"=w263) -> ("String"=w262:string)  [unwired: 9 in, 1 out]
                n162 = Unbundle(w261) -> (w257:string[])
                n163 = Match First String(2:w257, 3:w262) -> (0:w258:i32)  [unwired: 1 out]
                n164 = property on="Test Ring" class="Ring (strict)"("Value"=w258, "Strings []"=w257) -> ()  [unwired: 2 in, 2 out]
                n165 = property on="Test Ring" class="Ring (strict)"("Visible"=TRUE) -> ()  [unwired: 2 in, 2 out]
                n166 = property on="Test Slider" class="Slide (strict)"("Visible"=FALSE) -> ()  [unwired: 2 in, 2 out]
              }
              frame "Color Enable  **" {
                n167 = Index Array(array=w269, index=4) -> (element=w270:cluster{string[]})
                n168 = call <vilib>:"NT Read String.vi"("Name"=w272) -> ("String"=w271:string)  [unwired: 9 in, 1 out]
                n169 = Unbundle(w270) -> (w266:string[])
                n170 = Match First String(2:w266, 3:w271) -> (0:w267:i32)  [unwired: 1 out]
                n171 = property on="Test Ring" class="Ring (strict)"("Value"=w267, "Strings []"=w266) -> ()  [unwired: 2 in, 2 out]
                n172 = property on="Test Ring" class="Ring (strict)"("Visible"=TRUE) -> ()  [unwired: 2 in, 2 out]
                n173 = property on="Test Slider" class="Slide (strict)"("Visible"=FALSE) -> ()  [unwired: 2 in, 2 out]
              }
              frame Default {
                n174 = property on="Test Ring" class="Ring (strict)"("Visible"=FALSE) -> ()  [unwired: 2 in, 2 out]
                n175 = property on="Test Slider" class="Slide (strict)"("Visible"=FALSE) -> ()  [unwired: 2 in, 2 out]
              }
              frame "Brightness  **", "Color Level  **", "Compression  **", "FPS  **", "Sharpness  **" {
                n176 = call <vilib>:"NT Read Number.vi"("Name"=w278) -> ("Numeric"=w277:dbl)  [unwired: 9 in, 1 out]
                n177 = local write "Test Slider"(w277) -> ()
                n178 = property on="Test Slider" class="Slide (strict)"("Visible"=TRUE, "Scale.Maximum"=100.0 ("Scale.Range:Maximum")) -> ()  [unwired: 2 in, 2 out]
                n179 = property on="Test Ring" class="Ring (strict)"("Visible"=FALSE) -> ()  [unwired: 2 in, 2 out]
              }
            }
          }
        }
        n180 = property on="Progress" class="Clust (strict)"("Visible"=FALSE) -> ()  [unwired: 2 in, 2 out]
      }
      event "Test Name": Mouse Enter {
        # "Populate the ring with the list of tests"
        n181 = event-data() -> ()  [unwired: 1 in, 1 out]
        n182 = call <vilib>:"NT Read String Array.vi"("Name"="TestMode/TestList") -> ("String Array"=w286:string[])  [unwired: 9 in, 1 out]
        n183 = Build Array (concatenate)("Select the test to run...", w286) -> (w285:string[])
        n184 = property on="Test Name" class="Ring (strict)"("Strings []"=w285) -> ()  [unwired: 2 in, 2 out]
      }
      event "Test Name": Value Change {
        w288 = FALSE ("Visible")
        # "Tell the robot the test name to run"
        n185 = event-data() -> ("NewVal"=w292:u16)  [unwired: 1 in]
        n186 = property on="Test Name" class="Ring (strict)"() -> ("Strings []"=w293:string[])  [unwired: 2 in, 2 out]
        n187 = local write "Progress"(T5 {"Test Progress"=0, "Test Progress Text"=""} ("Progress")) -> ()
        n188 = Index Array(array=w293, index=w292) -> (element=w291:string)
        n189 = call <vilib>:"NT Write String.vi"("String"=w291, "Name"="TestMode/TestName") -> ()  [unwired: 9 in, 1 out]
        n190 = property on="Progress" class="Clust (strict)"("Visible"=TRUE) -> ()  [unwired: 2 in, 2 out]
        n191 = property on="Motor" class="Clust (strict)"("Visible"=w288) -> ()  [unwired: 2 in, 2 out]
        n192 = property on="Test Slider" class="Slide (strict)"("Visible"=w288) -> ()  [unwired: 2 in, 2 out]
        n193 = property on="On/Off" class="Bool (strict)"("Visible"=w288) -> ()  [unwired: 2 in, 2 out]
        n194 = property on="Rev/Fwd" class="Clust (strict)"("Visible"=w288) -> ()  [unwired: 2 in, 2 out]
        n195 = property on="Test Ring" class="Ring (strict)"("Visible"=w288) -> ()  [unwired: 2 in, 2 out]
      }
      event "Listbox": Double Click {
        # "Shift clears all"
        # "Update symbols on the listbox"
        n196 = event-data() -> ("PlatMods.Shift"=w296:bool, "Row"=w298:i32)  [unwired: 1 in]
        n197 = case shown="True" w296 {
          tunnel: w298 -> [w302 _]
          tunnel: 1 -> [w301 _]
          frame False {
            n198 = property on="Listbox" class="LstBox (strict)"() -> ("Item Symbols"=w300:i32[])  [unwired: 2 in, 2 out]
            n199 = Replace Array Subset(array=w300, new element=w301, index=w302) -> (w299:i32[])
            n200 = property on="Listbox" class="LstBox (strict)"("Item Symbols"=w299) -> ()  [unwired: 2 in, 2 out]
          }
          frame True {
            w303 = 0 ("Top Row")
            n201 = property on="Listbox" class="LstBox (strict)"() -> ("Number of Rows"=w305:u32)  [unwired: 2 in, 2 out]
            n202 = Initialize Array(0, w305) -> (w304:i32[])
            n203 = property on="Listbox" class="LstBox (strict)"("Top Row"=w303, "Value"=w303, "Item Symbols"=w304) -> ()  [unwired: 2 in, 2 out]
          }
        }
      }
      event "Listbox": Key Down {
        # "Update symbols on the listbox\nLeft and right keys check and uncheck"
        n204 = event-data() -> ("VKey"=w309:T16)  [unwired: 1 in]
        n205 = case shown="\"Left\", \"Right\"" w309 {
          selector: w309 -> [w314 _]
          tunnel: eventvkey."Left" ("VKey") -> [w312 _]
          frame "Left", "Right" {
            n206 = Equal?(x=w312, y=w314) -> (x = y?=w313:bool)
            n207 = Select(t=0, s=w313, f=1) -> (s? t:f=w315:i32)
            n208 = property on="Listbox" class="LstBox (strict)"() -> ("Item Symbols"=w318:i32[])  [unwired: 2 in, 2 out]
            n209 = Replace Array Subset(array=w318, new element=w315, index="Listbox") -> (w317:i32[])
            n210 = property on="Listbox" class="LstBox (strict)"("Item Symbols"=w317) -> ()  [unwired: 2 in, 2 out]
          }
          frame Default {
          }
        }
      }
      event "DB Camera Config": Value Change {
        # "Show or hide the cluster of controls, store in ini file"
        n211 = event-data() -> ("NewVal"=w322:bool)  [unwired: 1 in]
        n212 = case shown="False" w322 {
          tunnel: w321 -> [w331 _]
          tunnel: [w324 w342] -> w320
          tunnel: w319 -> [w323 w342]
          frame False {
            w338 = "Camera"
            w341 = FALSE ("Visible")
            n213 = local read "Camera Settings"() -> (w330:T3)
            n214 = Index Array(array=w331) -> (element=w334:cluster{string[]})  [unwired: 1 in]
            n215 = Unbundle(w330) -> ("Frame Rate"=w329:i32, "Compression"=w328:i32, "Size"=w332:u16)
            n216 = Unbundle(w334) -> (w333:string[])
            n217 = Index Array(array=w333, index=w332) -> (element=w327:string)
            n218 = call-poly <vilib>:"Write Key.vi"("section"=w338, "value"=w327, "key"="Size", "refnum"=w323) -> ("refnum out"=w340:T14)  [unwired: 2 in, 5 out]
            n219 = call-poly <vilib>:"Write Key.vi"("section"=w338, "value"=w329, "key"="FrameRate", "refnum"=w340) -> ("refnum out"=w339:T14)  [unwired: 1 in, 6 out]
            n220 = property on="Camera Settings" class="Clust (strict)"("Visible"=w341) -> ()  [unwired: 2 in, 2 out]
            n221 = local write "DB Camera Config"(w341) -> ()
            n222 = call-poly <vilib>:"Write Key.vi"("section"=w338, "value"=w328, "key"="Compression", "refnum"=w339) -> ("refnum out"=w325:T14)  [unwired: 1 in, 6 out]
            n223 = call <vilib>:"Close Config Data.vi"("refnum"=w325) -> ("file path"=w326:path)  [unwired: 2 in, 8 out]
            n224 = call <vilib>:"Open Config Data.vi"("configuration file path"=w326) -> ("refnum"=w324:T14)  [unwired: 8 in, 2 out]
          }
          frame True {
            n225 = property on="Camera Settings" class="Clust (strict)"("Visible"=TRUE) -> ()  [unwired: 2 in, 2 out]
          }
        }
      }
      event "Camera Settings": Value Change {
        # "Update summary string when any elements of DB camera change"
        n226 = event-data() -> ("NewVal"=w355:T3)  [unwired: 1 in]
        n227 = Index Array(array=w351) -> (element=w350:cluster{string[]})  [unwired: 1 in]
        n228 = Unbundle(w355) -> ("Frame Rate"=w346:i32, "Compression"=w345:i32, "Size"=w348:u16)
        n229 = Unbundle(w350) -> (w349:string[])
        n230 = Index Array(array=w349, index=w348) -> (element=w347:string)
        n231 = Format Into String(format string="%s   %dfps   %d%%", w347, w346, w345) -> (resulting string=w352:string)  [unwired: 2 in, 1 out]
        n232 = Build Array(w352) -> (w353:string[])
        n233 = property on="DB Camera Config" class="Bool (strict)"("Strings [4]"=w353) -> ()  [unwired: 2 in, 2 out]
      }
      event "Motor.Enable": Value Change {
        # "When the test mode otor enable helper is set, update that\ntree row item's value"
        n234 = event-data() -> ("NewVal"=w361:bool)  [unwired: 1 in]
        n235 = Unbundle("Motor") -> ("Value"=w360:dbl)  [unwired: 1 out]
        n236 = Select(t=w360, s=w361, f=0.0) -> (s? t:f=w358:dbl)
        n237 = call <vilib>:"NT Write Number.vi"("Numeric"=w358, "Name"=w357) -> ()  [unwired: 9 in, 1 out]
      }
      event "Test Slider": Value Change {
        # "When the test mode slider helper is set, update that\ntree row item's value"
        n238 = event-data() -> ("NewVal"=w364:dbl)  [unwired: 1 in]
        n239 = call <vilib>:"NT Write Number.vi"("Numeric"=w364, "Name"=w365) -> ()  [unwired: 9 in, 1 out]
      }
      event "On/Off": Value Change {
        # "When the test mode on/off helper value is set, update that\ntree row item's value"
        n240 = event-data() -> ("NewVal"=w369:bool)  [unwired: 1 in]
        n241 = Boolean To (0,1)(Boolean=w369) -> (0, 1=w368:i16)
        n242 = call <vilib>:"NT Write Number.vi"("Numeric"=w368, "Name"=w367) -> ()  [unwired: 9 in, 1 out]
      }
      event "Rev/Fwd": Value Change {
        # "When the test mode helper value for relays is set, update that\ntree row item's value"
        n243 = event-data() -> ("NewVal.Forward"=w377:bool, "NewVal.Reverse"=w376:bool)  [unwired: 1 in]
        n244 = Boolean To (0,1)(Boolean=w377) -> (0, 1=w373:i16)
        n245 = Boolean To (0,1)(Boolean=w376) -> (0, 1=w375:i16)
        n246 = Negate(x=w375) -> (-x=w374:i16)
        n247 = Add(x=w373, y=w374) -> (x+y=w372:i16)
        n248 = call <vilib>:"NT Write Number.vi"("Numeric"=w372, "Name"=w371) -> ()  [unwired: 9 in, 1 out]
      }
      event "Test Ring": Value Change {
        # "When a test mode helper value is selected from the ring,\nset the tree item's variable to the string value"
        n249 = event-data() -> ("NewVal"=w381:u16)  [unwired: 1 in]
        n250 = property on="Test Ring" class="Ring (strict)"() -> ("Strings []"=w382:string[])  [unwired: 2 in, 2 out]
        n251 = Index Array(array=w382, index=w381) -> (element=w380:string)
        n252 = call <vilib>:"NT Write String.vi"("String"=w380, "Name"=w379) -> ()  [unwired: 9 in, 1 out]
      }
      event "Rec Mode": Value Change {
        # "Update globals for recording mode and path to read log from.\nClear when logging and let NetworkTables set path for vision to\nuse."
        n253 = event-data() -> ("NewVal"=w392:enum32{"Stop", "Record", "Playback"})  [unwired: 1 in]
        n254 = global write "WPI_DashboardLogging Global.vi" "Logging Filename"(path "") -> ()
        n255 = case shown="\"Playback\"" w392 {
          tunnel: w391 -> [_ w394 w402]
          tunnel: [_ _ w401] -> w388
          tunnel: [_ _ w400] -> _
          tunnel: w386 -> [_ _ w398]
          tunnel: cluster{i32, i32} {-250, 170} -> [_ _ w397]
          tunnel: [_ _ T17 {"Image Size"=TRUE, "Image Type"=TRUE, "Pixel Value"=TRUE, "ROI Information"=TRUE, "Zoom Factor"=FALSE} ("Image Information Shown:All Elements")] -> w384
          tunnel: [_ _ TRUE ("Zoom Factor")] -> w383
          frame Default {
          }
          frame "Stop", "Record" {
            # "Place Window too"
            n256 = invoke class="VI" method="FP.Close"(reference=w394) -> (reference out=w393:refnum<vi>)  [unwired: 2 in, 2 out]
            n257 = invoke class="VI" method="Abort VI"(reference=w393) -> ()  [unwired: 2 in, 3 out]
          }
          frame "Playback" {
            n258 = call "Open Playback Panel.vi"("Offset"=w397, "DB VI Ref"=w398, "Playback in"=w402) -> ("Playback out"=w399:refnum<vi>)  [unwired: 8 in]
            n259 = register-events(w399) -> (reference out=w401:refnum<event-registration>, error out=w400:errorcluster)  [unwired: 2 in]
          }
        }
        n260 = global write "WPI_DashboardLogging Global.vi" "Recording"(w392) -> ()
        n261 = property on="Camera Image" class="ImageControl"("Image Information Shown"=w384, "Image Information Visible"=w383) -> ()  [unwired: 2 in, 2 out]
        n262 = call <vilib>:"WPI_DashboardNT Log FieldName Cache.vi"("Operation"=enum16{"Lookup/Add", "Index", "Clear"}."Clear") -> ()  [unwired: 8 in, 3 out]
      }
      event Panel Close {
        w403 = enum32{"Stop", "Record", "Playback"}."Stop" ("Rec Mode")
        # "Playback window has been closed, abort"
        n263 = event-data() -> ()  [unwired: 1 in, 4 out]
        n264 = local write "Rec Mode"(w403) -> ()
        n265 = global write "WPI_DashboardLogging Global.vi" "Recording"(w403) -> ()
      }
      event Panel Close {
        # "Abort playback window and ourself"
        n266 = event-data() -> ()  [unwired: 1 in, 4 out]
        n267 = invoke class="VI" method="FP.Close"(reference=w408) -> (reference out=w407:refnum<vi>)  [unwired: 2 in, 2 out]
        n268 = invoke class="VI" method="Abort VI"(reference=w407) -> (error out=w406:errorcluster)  [unwired: 2 in, 2 out]
        n269 = invoke class="VI" method="Abort VI"(error in=w406) -> ()  [unwired: 2 in, 3 out]
      }
      event "Vision": Value Change {
        # "Enable/Disable Compression slider.\nHW USB is hard-coded into the camera"
        n270 = event-data() -> ("NewVal"=w414:u16)  [unwired: 1 in]
        n271 = Equal?(x=w414, y=u32 2 ("milliseconds to wait")) -> (x = y?=w412:bool)
        n272 = Select(t=T18."Disabled and Grayed Out" ("Disabled"), s=w412, f=T18."Enabled" ("Disabled")) -> (s? t:f=w409:T18)
        n273 = property on="Compression" class="Slide (strict)"("DisabledEnum"=w409) -> ()  [unwired: 2 in, 2 out]
      }
    }
  }
  n274 = while {
    tunnel: w38 -> [w417]
    i -> [w420]
    stop <- FALSE stop-if-true
    n275 = Wait (ms)(milliseconds to wait=u32 100) -> ()  [unwired: 1 out]
    n276 = case shown="\"Playback\"" "Rec Mode" {
      tunnel: w420 -> [_ _ w435]
      tunnel: [u32 2829099 ("Base Color") u32 11141120 ("Target Color") w424] -> w416
      frame "Stop", Default {
        # "Reset the color, extra updates don't cost much"
      }
      frame "Record" {
      }
      frame "Playback" {
        # "Playback"
        n277 = Quotient & Remainder(x=w435, y=u32 50 ("milliseconds to wait")) -> (x-y*floor(x/y)=w431:u32)  [unwired: 1 out]
        n278 = Divide(x=w431, y=u32 50 ("milliseconds to wait")) -> (x/y=w428:dbl)
        n279 = Multiply(x=6.283185307179586, y=w428) -> (x*y=w433:dbl)
        n280 = Sine(x=w433) -> (sin(x)=w432:dbl)
        n281 = Absolute Value(x=w432) -> (abs(x)=w425:dbl)
        n282 = call "Interpolate RGB Color.vi"("Proportion"=w425, "Target Color"=u32 30976, "Base Color"=u32 2829099) -> ("Result Color"=w424:u32)  [unwired: 8 in]
      }
    }
    n283 = property class="Pane"(reference=w417, "PaneColor"=w416) -> ()  [unwired: 1 in, 2 out]
  }
  n284 = TCP Create Listener(10:u16 1741 ("timeout ms (25000)")) -> (3:w1:refnum<k5>)  [unwired: 4 in, 2 out]
  n285 = while {
    tunnel: w1 -> [w437]
    stop <- FALSE stop-if-true
    n286 = TCP Wait On Listener(11:w437) -> (4:w436:refnum<k5>)  [unwired: 3 in, 4 out]
    n287 = local write "TCP"(w436) -> ()
  }
  n288 = property on="On/Off" class="Bool (strict)"("Visible"=w6) -> ()  [unwired: 2 in, 2 out]
  n289 = property on="Motor" class="Clust (strict)"("Visible"=w6) -> ()  [unwired: 2 in, 2 out]
  n290 = property on="Progress" class="Clust (strict)"("Visible"=w6) -> ()  [unwired: 2 in, 2 out]
  n291 = property on="Test Ring" class="Ring (strict)"("Visible"=w6) -> ()  [unwired: 2 in, 2 out]
  n292 = property on="Rev/Fwd" class="Clust (strict)"("Visible"=w6) -> ()  [unwired: 2 in, 2 out]
  n293 = property on="Camera Settings" class="Clust (strict)"("Visible"=w6) -> ()  [unwired: 2 in, 2 out]
  n294 = local write "DB Camera Config"(w6) -> ()
  n295 = global write "WPI_DashboardLogging Global.vi" "Recording"(w32) -> ()
  n296 = local write "Rec Mode"(w32) -> ()
